vi "cmdCode2Text.vi"(3 "error in (no error)":errorcluster caption="错误输入（无错误）", 4 "CommandCode":string) -> (0 "error out":errorcluster caption="错误输出", 1 "CommandText":T1)   [LabVIEW 2010]
uses:
  OutputDataFormat.ctl
  VarableID.ctl
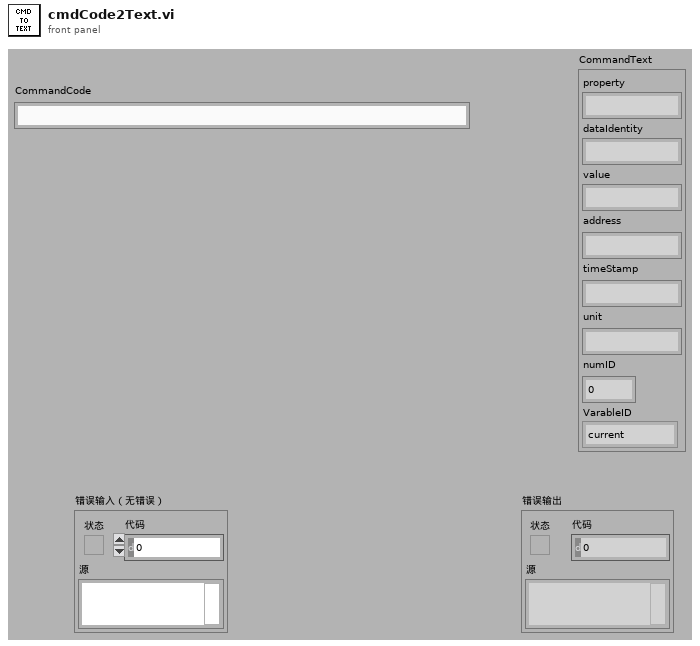
[diagram p1: front panel]
types:
  T1 = typedef "OutputDataFormat.ctl" = cluster{"property":string, "dataIdentity":string, "value":string, "address":string, "timeStamp":string, "unit":string, "numID":i32, "VarableID":T2}
  T2 = typedef "VarableID.ctl" = enum16{"current", "power", "PF", "voltage"}
  T3 = cluster{"address":string, "controlCode":string, "dataLength":dbl, "dataSection":string, "checkCode":string}
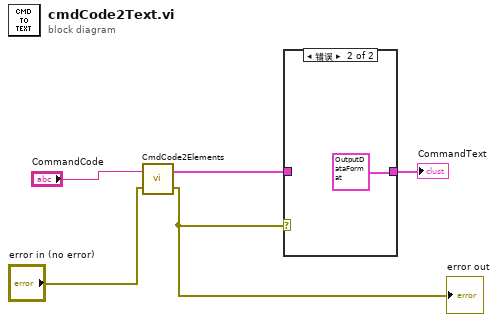
[diagram p0: block diagram]
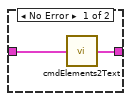
[diagram p2: hidden frame]
diagram:
  n1 = call "CmdCode2Elements.vi"("error in (no error)"="error in (no error)", "CommandCode"="CommandCode") -> ("error out"=w1:errorcluster, "Elements"=w5:T3)
  "error out" <- w1
  n2 = case shown="错误" w1 {
    tunnel: w5 -> [w7 _]
    tunnel: [w6 T1 {"property"="", "dataIdentity"="", "value"="", "address"="", "timeStamp"="", "unit"="", "numID"=0, "VarableID"=enum."current"} ("CommandText")] -> w3
    frame No Error {
      n3 = call "cmdElements2Text.vi"("CodeElements"=w7) -> ("CommandText"=w6:T1)
    }
    frame Error {
    }
  }
  "CommandText" <- w3
